vi "ICA_17_Potluri.vi"() -> ()   [LabVIEW 2016]
uses:
  <vilib>/NXT/Block Support/NXT_OutputPort.ctl
  <vilib>/NXT/Dual Mode Library/Sensors/EV3_Color_Reflect.vi
  <vilib>/NXT/Dual Mode Library/Sensors/EV3_Ultrasonic_CM.vi
  <vilib>/NXT/NXTIO Xnodes/NXTIONodeSubVIs/LEGOMoveAllMotors.vi
  <vilib>/NXT/NXTIO Xnodes/NXTIONodeSubVIs/NXTMotorRunDistance.vi
  <vilib>/NXT/NXTIO Xnodes/NXTIONodeSubVIs/LEGOStopAllMotors.vi
  <vilib>/NXT/NXTIO Xnodes/NXTIOXNode/NXTIO.xnode
  <vilib>/NXT/Subs/LVHSConnector.ctl
  <vilib>/NXT/NXTIO Xnodes/AddressXNode/NXTIOAddress.xnode
  <vilib>/NXT/LegoClasses/BrickReference/BrickReference.lvclass
panel:
  out "Numeric 4":dbl
  out "Numeric 3":dbl
  out "Numeric 2":dbl
  out "Numeric":dbl
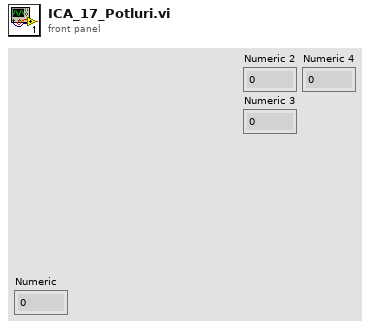
[diagram p1: front panel]
types:
  T1 = typedef "LVHSConnector.ctl" = refnum<class "BrickReference.lvclass">
  T2 = typedef "NXT_OutputPort.ctl" = u8
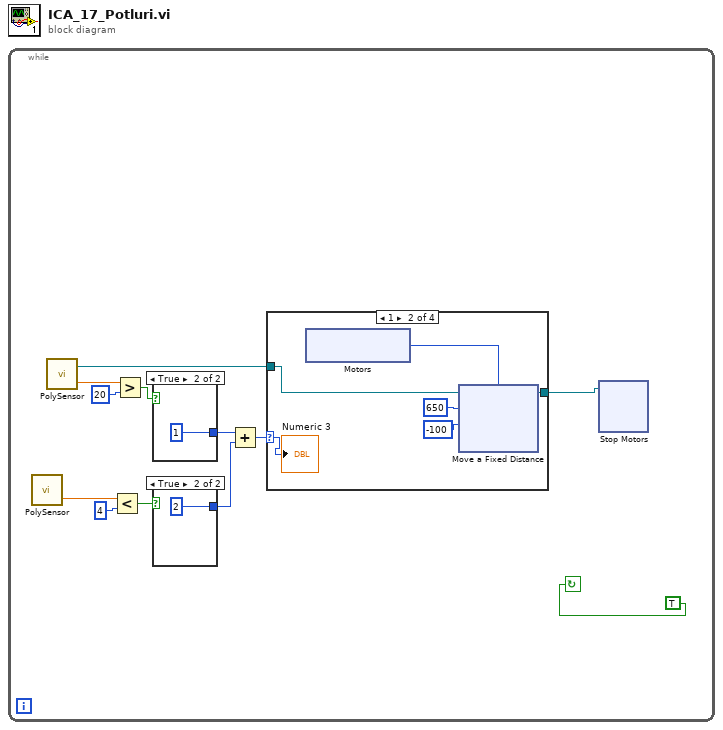
[diagram p0: block diagram]
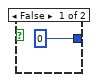
[diagram p2: hidden frame]
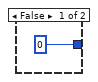
[diagram p3: hidden frame]
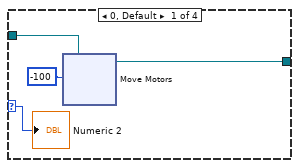
[diagram p4: hidden frame]
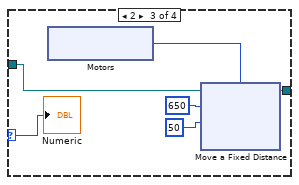
[diagram p5: hidden frame]
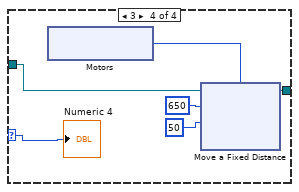
[diagram p6: hidden frame]
diagram:
  n1 = while {
    stop <- TRUE continue-if-true
    n2 = call-poly <vilib>:"PolySensor.vi"() -> ("Scaled Value"=w11:sgl)  [unwired: 3 in, 1 out]
    n3 = call-poly <vilib>:"PolySensor.vi"() -> ("Centimeters"=w8:sgl, "NXT/EV3"=w2:T1)  [unwired: 3 in]
    n4 = Less?(x=w11, y=4) -> (x < y?=w6:bool)
    n5 = Greater?(x=w8, y=20) -> (0:w7:bool)
    n6 = case shown="True" w7 {
      tunnel: [0 1] -> w4
      frame False {
      }
      frame True {
      }
    }
    n7 = case shown="True" w6 {
      tunnel: [0 2] -> w5
      frame False {
      }
      frame True {
      }
    }
    n8 = Add(x=w4, y=w5) -> (x+y=w3:i32)
    n9 = case shown="1" w3 {
      selector: w3 -> [w21 w30 w47 w64]
      tunnel: w2 -> [w23 w33 w49 w65]
      tunnel: [w20 w29 w46 w63] -> w1
      frame 0, Default {
        n10 = xnode "Move Motors"("Power/Speed 1"=-100, "NXT/EV3"=w23) -> ("NXT/EV3"=w20:T1)  [unwired: 1 in]
        "Numeric 2" <- w21
      }
      frame 1 {
        n11 = xnode "Motors"() -> ("Motor"=w34:T2)
        n12 = xnode "Move a Fixed Distance"("Speed 1"=-100, "Distance 1"=650, "Motors"=w34, "NXT/EV3"=w33) -> ("NXT/EV3"=w29:T1)
        "Numeric 3" <- w30
      }
      frame 2 {
        n13 = xnode "Motors"() -> ("Motor"=w48:T2)
        n14 = xnode "Move a Fixed Distance"("Speed 1"=50, "Distance 1"=650, "Motors"=w48, "NXT/EV3"=w49) -> ("NXT/EV3"=w46:T1)
        "Numeric" <- w47
      }
      frame 3 {
        n15 = xnode "Motors"() -> ("Motor"=w66:T2)
        n16 = xnode "Move a Fixed Distance"("Speed 1"=50, "Distance 1"=650, "Motors"=w66, "NXT/EV3"=w65) -> ("NXT/EV3"=w63:T1)
        "Numeric 4" <- w64
      }
    }
    n17 = xnode "Stop Motors"("NXT/EV3"=w1) -> ()  [unwired: 1 in, 1 out]
  }
